vi "Module Not Stopped--error.vi"() -> (0 "error out":errorcluster)   [LabVIEW 2021, in "RT-TDMS-Logging.lvlib"]
doc: "Outputs an error cluster containing a custom error code indicating the Stop Module VI timed out while waiting for the module main VI to stop.\n_____\nBased on DQMH Project Template 7.0.1.1316."
uses:
  RT-TDMS-Logging.lvlib
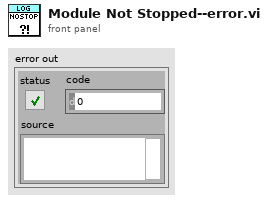
[diagram p1: front panel]
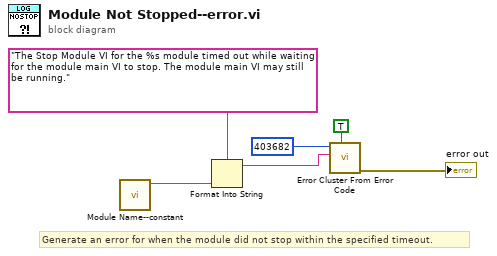
[diagram p0: block diagram]
diagram:
  # "Generate an error for when the module did not stop within the specified timeout."
  n1 = call "Module Name--constant.vi"() -> ("Module Name"=w2:string)  [unwired: 11 in]
  n2 = Format Into String(format string="The Stop Module VI for the %s module timed out while waiting for the module main VI to stop. The module main VI may still be running.", w2) -> (resulting string=w4:string)  [unwired: 2 in, 1 out]
  n3 = call <vilib>:"Error Cluster From Error Code.vi"("show call chain? (False)"=TRUE, "error message (\"\")"=w4, "error code (0)"=403682) -> ("error out"=→"error out":errorcluster)  [unwired: 6 in]
